vi "WPI_DashboardRetrieve Command Params.vi"(11 "RPC Buffer":string) -> (3 "Param Info":string[][](array[string]))   [LabVIEW 2017]
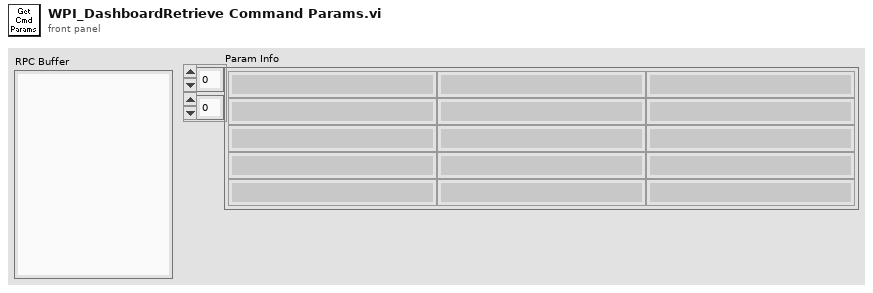
[diagram p1: front panel]
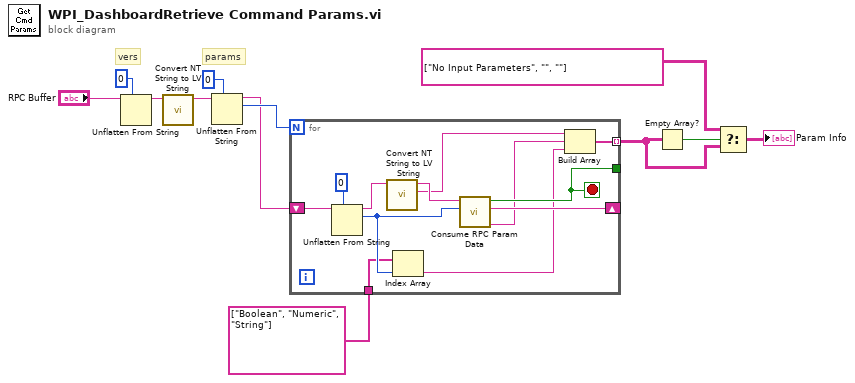
[diagram p0: block diagram]
diagram:
  # "params"
  # "vers"
  n1 = Unflatten From String(type=u8 0 ("bytes to read"), binary string="RPC Buffer") -> (rest of the binary string=w7:string)  [unwired: 3 in, 2 out]
  n2 = call <vilib>:"Convert NT String to LV String.vi"("Buffer in"=w7) -> ("Remaining String"=w9:string)  [unwired: 8 in, 2 out]
  n3 = Unflatten From String(type=u8 0 ("bytes to read"), binary string=w9) -> (rest of the binary string=w3:string, value=w4:u8)  [unwired: 3 in, 1 out]
  n4 = for {
    N: w4 -> [_]
    shift-right: [w21] -> _
    shift-left: w3 -> [w23]
    tunnel: [w20] -> _
    tunnel: string[] ["Boolean", "Numeric", "String"] -> [w17]
    tunnel: [w14] -> w1 mode=indexing
    stop <- w20 stop-if-true
    n5 = Unflatten From String(type=u8 0 ("bytes to read"), binary string=w23) -> (rest of the binary string=w22:string, value=w18:u8)  [unwired: 3 in, 1 out]
    n6 = call <vilib>:"Convert NT String to LV String.vi"("Buffer in"=w22) -> ("String Contents"=w13:string, "Remaining String"=w19:string)  [unwired: 8 in, 1 out]
    n7 = Index Array(array=w17, index=w18) -> (element=w16:string)
    n8 = call <vilib>:"Consume RPC Param Data.vi"("type"=w18, "RPC String in"=w19) -> ("Value String"=w15:string, "string out"=w21:string, "Issue"=w20:bool)  [unwired: 6 in, 1 out]
    n9 = Build Array(w13, w15, w16) -> (w14:string[])
  }
  n10 = Empty Array?(array=w1) -> (empty?=w10:bool)
  n11 = Select(t=string[][] [["No Input Parameters", "", ""]], s=w10, f=w1) -> (s? t:f=→"Param Info":string[][])
